vi "Write Data reduction.vi"(8 "error in (no error)":errorcluster, 10 "Data reduction":T1={"Clip time"=FALSE, "Tiime 0"=0.0, "Time 1"=0.0, "Maximum data points"=1, "Decimation method"=enum."Min-Max"}, 11 "Plot in":refnum<class "Plot.lvclass">) -> (0 "error out":errorcluster, 3 "Plot out":refnum<class "Plot.lvclass">)   [LabVIEW 2018, in "Plot.lvclass"]
uses:
  Plot.lvclass
  NHMFL_Core/Libraries/File/Controls/Data reduction.ctl
  Plot.lvclass/Plot.ctl
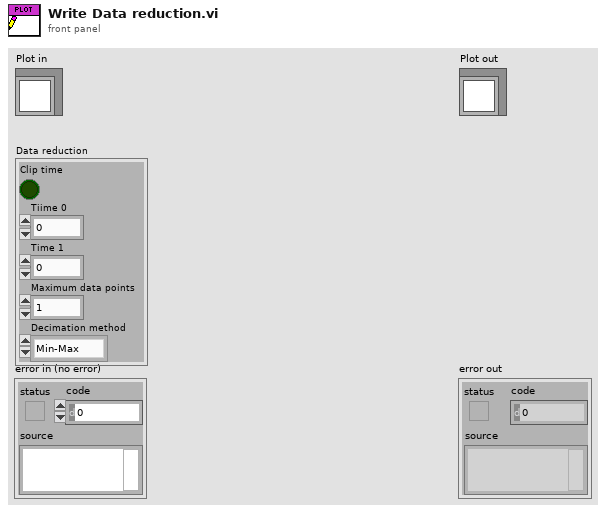
[diagram p1: front panel]
types:
  T1 = typedef "Data reduction.ctl" = cluster{"Clip time":bool, "Tiime 0":dbl, "Time 1":dbl, "Maximum data points":i32, "Decimation method":enum16{"coerce", "linear", "spline", "Min-Max", "Average"}}
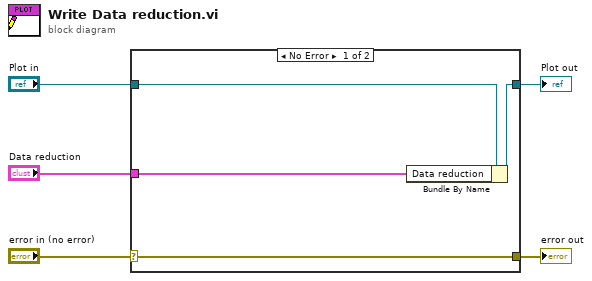
[diagram p0: block diagram]
diagram:
  n1 = case shown="No Error" "error in (no error)" {
    selector: "error in (no error)" -> [w9 w10]
    tunnel: [w9 w10] -> w4
    tunnel: [w7 w11] -> w2
    tunnel: "Plot in" -> [w8 w11]
    tunnel: "Data reduction" -> [w6 _]
    frame No Error {
      n2 = Bundle By Name(cluster=w8, "Data reduction"=w6) -> (w7:refnum<class "Plot.lvclass">)
    }
    frame Error {
    }
  }
  "error out" <- w4
  "Plot out" <- w2
